vi "WindSensorSampleSensorLoop.vi"   [LabVIEW 2018]
uses:
  WindSensorSampleSensorLoopData.ctl
  WindSensorSampleSensorLoopStates.ctl
  WindSensorSample.ctl
  WindSensorErrorSample.ctl
  WindSensorErrorCodes.ctl
  <vilib>/Platform/TimedLoop/XDataNode/timing_clust.ctl
  <vilib>/Platform/TimedLoop/XDataNode/nitl_modes.ctl
  <vilib>/Platform/TimedLoop/XDataNode/wakeup.ctl
  <vilib>/rvi/Emulation/niFpgaSctlEmulationGetInTimedLoop.vi
  <vilib>/rvi/Emulation/niFpgaEmulationReportErrorSimple.vi
  <vilib>/rvi/Emulation/niFpgaGetClockAttributes.vi
  <vilib>/rvi/Emulation/niFpgaCriticalErrorInLSC.vi
  <vilib>/rvi/Emulation/niFpgaEmulationIsFPGAContextNoSignature.vi
  <vilib>/rvi/FIFO/Fifo_Resource/nirvififoEmulationSetSize.vi
  <vilib>/rvi/DataTransferAndStorage/Container/Common/niFpgaContainerGetUniqueNameForEmu.vi
  <vilib>/rvi/FIFO/Fifo_Resource/nirviFifoEmulationQueueMgr.vi
  <instcachedir>/0/nirviFifoEmulationQueueMgr_E5CAEC123FF24DC58D834DCA3CDAA9B5.lvgen/nirviFifoEmulationQueueMgr_E5CAEC123FF24DC58D834DCA3CDAA9B5_001.vi
  <vilib>/rvi/Emulation/niFpgaProcessEmulError.vi
  <vilib>/rvi/Memory/Memory_Emulation/niFpgaMemoryEmulationCacheClearOnFirstRun.vi
  <vilib>/rvi/Memory/Memory_Emulation/nirvimemoryEmulationManagerCache_MakeExclusive.vi
  <vilib>/rvi/Memory/Memory_Emulation/niFpgaMemoryEmulationValidateCache.vi
  <vilib>/rvi/Memory/Memory_Emulation/nirvimemoryEmulationManagerCache_InsertValue.vi
  <vilib>/Utility/error.llb/Clear Errors.vi
  <vilib>/rvi/Memory/Memory_Emulation/nirvimemoryEmulationManagerCache_ReleaseExclusive.vi
  <vilib>/rvi/Memory/Memory_Emulation/nirvimemoryEmulationManagerCache_GetValue.vi
  <vilib>/rvi/Memory/Memory_Emulation/nirvimemoryEmulationManagerCache_SetValue.vi
  <vilib>/rvi/errors/niFpgaSetErrorForExecOnDevCompSimple.vi
  <vilib>/rvi/eio/common/nirviEmuReportErrorAndStop.vi
  <instcachedir>/0/nirviFifoEmulationQueueMgr_E5CAEC123FF24DC58D834DCA3CDAA9B5.lvgen/nirviFifoEmulationQueueMgr_E5CAEC123FF24DC58D834DCA3CDAA9B5_002.vi
  <vilib>/rvi/FIFO/Fifo_Resource/nirvififoEmulationDetermineInputValidOut.vi
  <vilib>/rvi/FIFO/Fifo_Resource/nirvififoEmulationCreateLock.vi
  <vilib>/rvi/FIFO/Fifo_Resource/nirvififoEmulationObtainLock.vi
  <vilib>/rvi/FIFO/Fifo_Resource/nirvififoEmulationReleaseLock.vi
  <vilib>/rvi/occurrence/nirviWaitOnOccurrenceBase.vi
  <vilib>/rvi/errors/nirviReportUnexpectedCaseInternalError.vi
  <vilib>/rvi/errors/nirviReportUnexpectedCaseInternalError (U32).vi
  <instcachedir>/0/nirviFifoEmulationQueueMgr_E5CAEC123FF24DC58D834DCA3CDAA9B5.lvgen/nirviFifoEmulationQueueMgr_E5CAEC123FF24DC58D834DCA3CDAA9B5_004.vi
  <instcachedir>/0/nirviFifoEmulationQueueMgr_E5CAEC123FF24DC58D834DCA3CDAA9B5.lvgen/nirviFifoEmulationQueueMgr_E5CAEC123FF24DC58D834DCA3CDAA9B5_026.vi
  <instcachedir>/0/nirviFifoEmulationQueueMgr_E5CAEC123FF24DC58D834DCA3CDAA9B5.lvgen/nirviFifoEmulationQueueMgr_E5CAEC123FF24DC58D834DCA3CDAA9B5_027.vi
  <vilib>/Platform/TimedLoop/XDataNode/XDataNode.xnode
  <vilib>/rvi/DataTransferAndStorage/Container/XNode/niFpgaContainer.xnode
  <vilib>/rvi/FIFO/Fifo_Resource/nirvififoEmulationGetNumberOfElementsToRead.vi
  <vilib>/rvi/DataTransferAndStorage/Register/Emulation/niFpgaRegisterEmulation.vi
  <vilib>/rvi/FIFO/Fifo_Resource/nirvififoEmulationWrite.vi
  <vilib>/rvi/FIFO/Fifo_Resource/nirvififoEmulationRead.vi
  <vilib>/Platform/TimedLoop/XDataNode/XDNodeRunTimeDep.lvlib
types:
  T1 = typedef "WindSensorSampleSensorLoopData.ctl" = cluster{"State":T2, "StateAfterRead":T2, "Timestamp":u64, "U16":u16, "Negative":bool, "SGL":i32, "Timeout":i32, "Sample":T3, "ErrorSample":T4, "PushSignature":bool, "IgnoreComa":bool}
  T2 = typedef "WindSensorSampleSensorLoopStates.ctl" = enum16{"WaitForData", "StartX", "EndX", "StartY", "EndY", "StartZ", "EndZ", "StartT", "EndT", "StartD", "EndD", "StartC", "EndC", "StartS", "EndS", "CheckSignature", "ReadSGL", "ReadU16", "ReadHexU16", "PrepareSample", "MoveSample", "ResponseUnknownError", "ResponseInvalidError", "ResponseTimeoutError", "ResponseSignatureError", "PrepareErrorCode", "MoveErrorCode", "ClearRxFIFO", "WaitForClearComplete"}
  T3 = typedef "WindSensorSample.ctl" = cluster{"Timestamp":u64, "TxBytes":u64, "RxBytes":u64, "TxFrames":u64, "RxFrames":u64, "X":i32, "Y":i32, "Z":i32, "Temperature":i32, "DiagnosticWord":u16, "Count":u8, "Signature":u16}
  T4 = typedef "WindSensorErrorSample.ctl" = cluster{"Timestamp":u64, "TxBytes":u64, "RxBytes":u64, "TxFrames":u64, "RxFrames":u64, "ErrorCode":T5}
  T5 = typedef "WindSensorErrorCodes.ctl" = enum16{"None", "ResponseUnknownError", "ResponseInvalidError", "ResponseTimeoutError", "ResponseSignatureError"}
  T6 = typedef "XDNodeRunTimeDep.lvlib/timing_clust.ctl" = cluster{"Expected End [f-1]":u64, "Actual End [f-1]":u64, "Finished Late? [f-1]":bool, "Expected End [i-1]":u64, "Actual End [i-1]":u64, "Finished Late? [i-1]":bool, "Expected Start [i]":u64, "Actual Start [i]":u64, "Expected Start [f]":u64, "Actual Start [f]":u64, "Source Name":string, "Structure Name":string, "Period":i64, "Deadline":i64, "Offset":i64, "Start":i64, "Priority":i32, "Timeout":i32, "Mode":T7, "Wakeup Reason":T8, "Error":errorcluster, "Source Type":string, "Secondary Source Type":string, "Global End Time":u64, "Global Start Time":u64, "Frame Duration":u64, "Iteration Duration":u64, "Assigned CPU":i32, "I/O Scan Engine Mode":u32}
  T7 = typedef "XDNodeRunTimeDep.lvlib/nitl_modes.ctl" = enum32{"No Change", "Process missed periods, maintain original phase", "Discard missed periods, maintain original phase", "Process missed periods, ignore original phase", "Discard missed periods, ignore original phase"}
  T8 = typedef "XDNodeRunTimeDep.lvlib/wakeup.ctl" = enum32{"Normal", "Aborted", "Asynchronous wakeup", "Timing source error", "Timed loop error", "Timeout"}
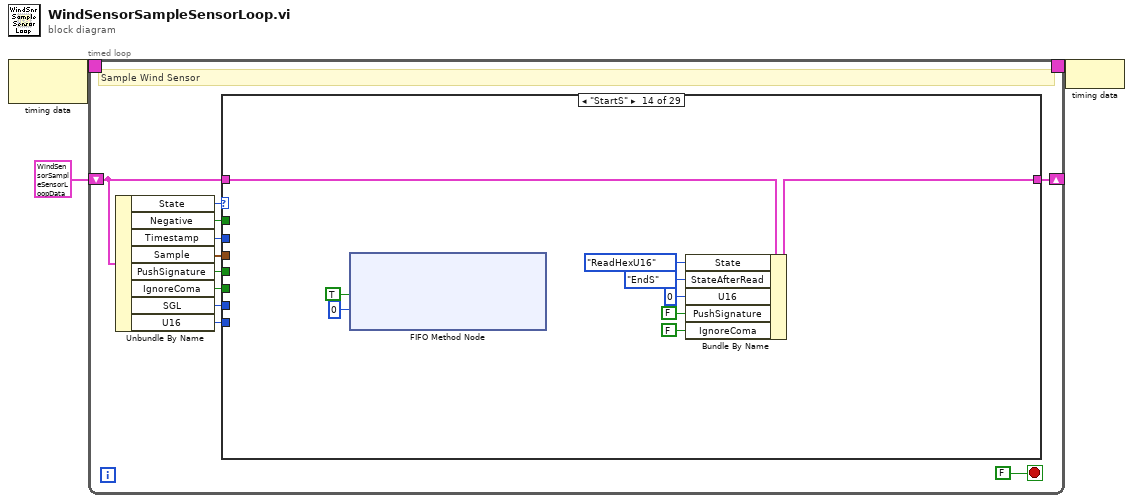
[diagram p0: block diagram]
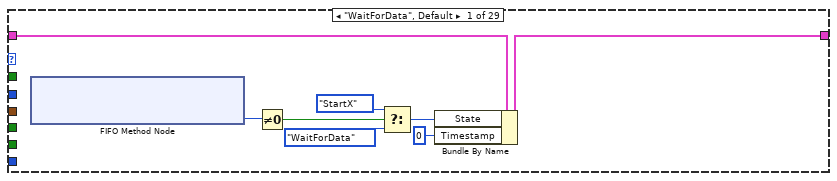
[diagram p2: hidden frame]
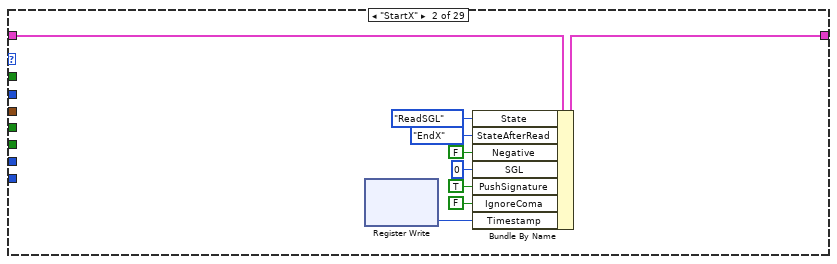
[diagram p3: hidden frame]
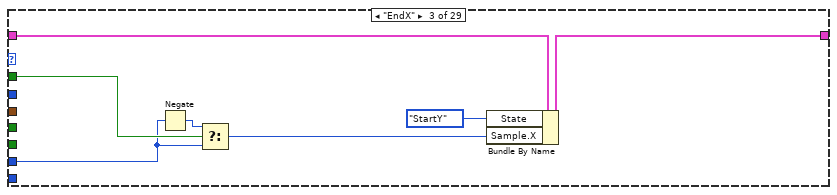
[diagram p4: hidden frame]
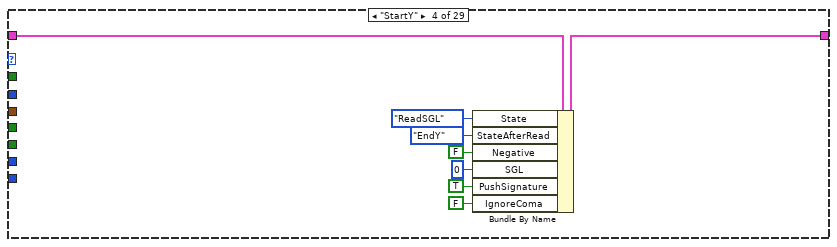
[diagram p5: hidden frame]
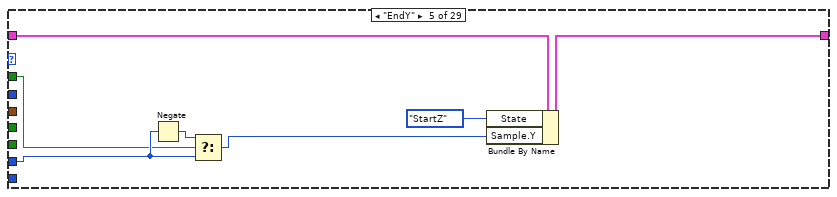
[diagram p6: hidden frame]
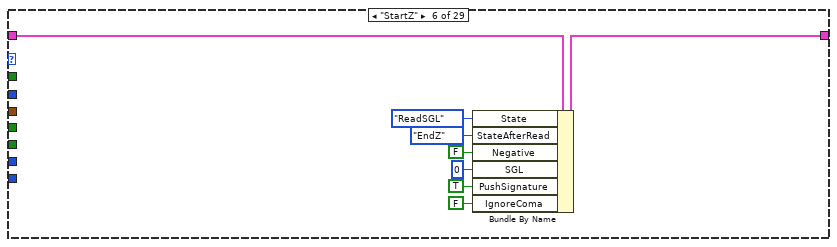
[diagram p7: hidden frame]
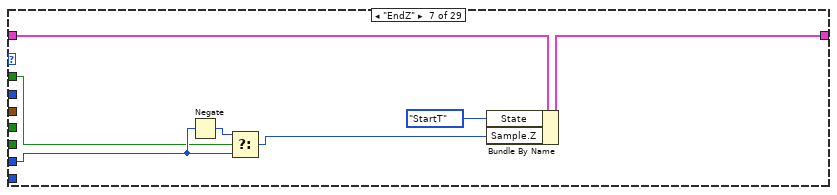
[diagram p8: hidden frame]
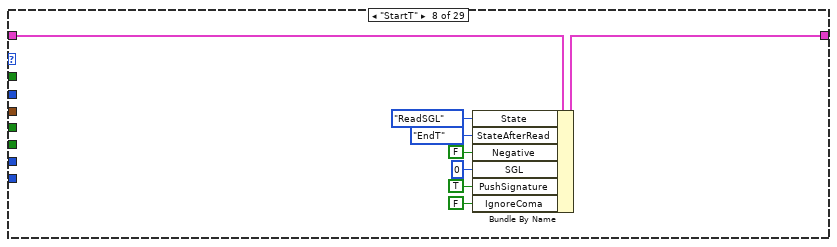
[diagram p9: hidden frame]
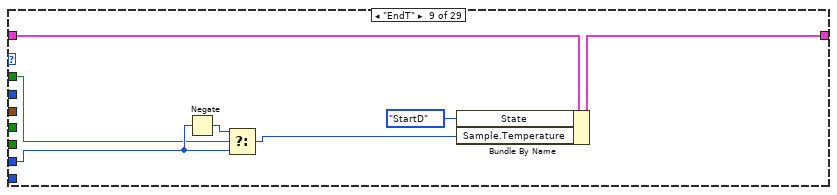
[diagram p10: hidden frame]
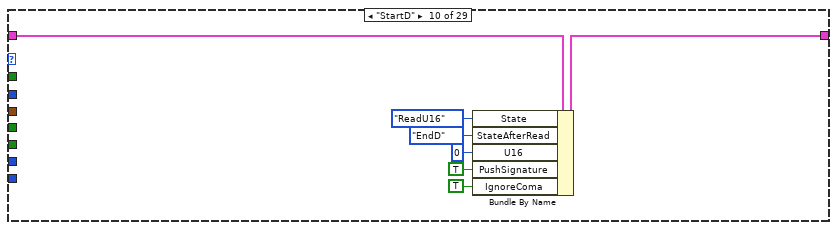
[diagram p11: hidden frame]
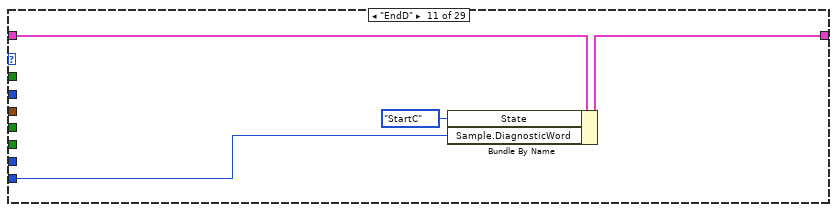
[diagram p12: hidden frame]
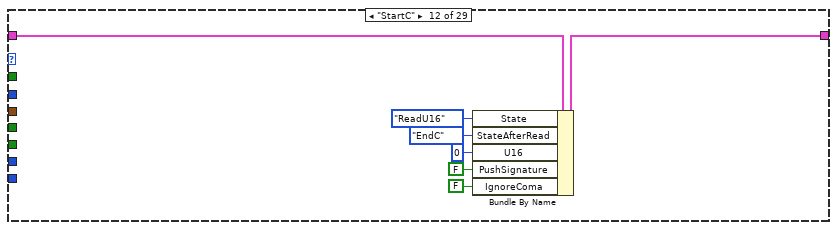
[diagram p13: hidden frame]
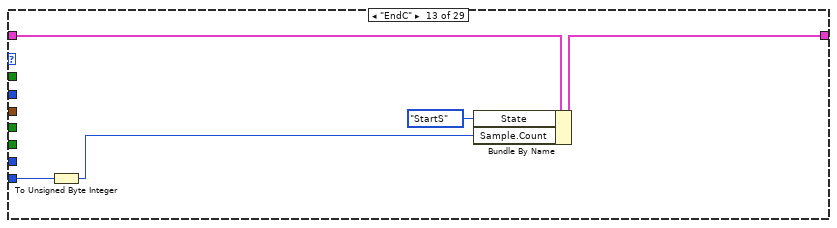
[diagram p14: hidden frame]
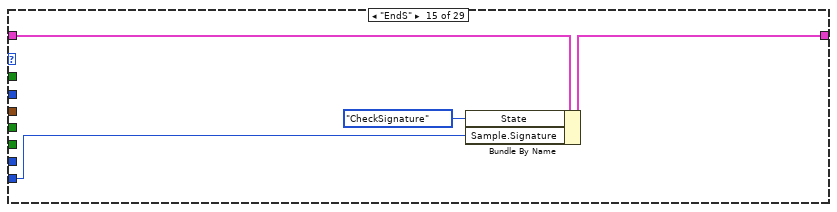
[diagram p15: hidden frame]
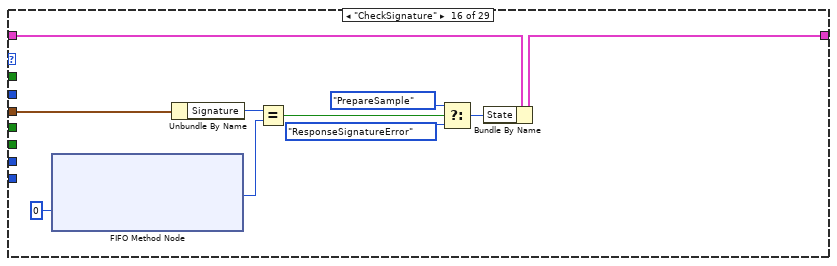
[diagram p16: hidden frame]
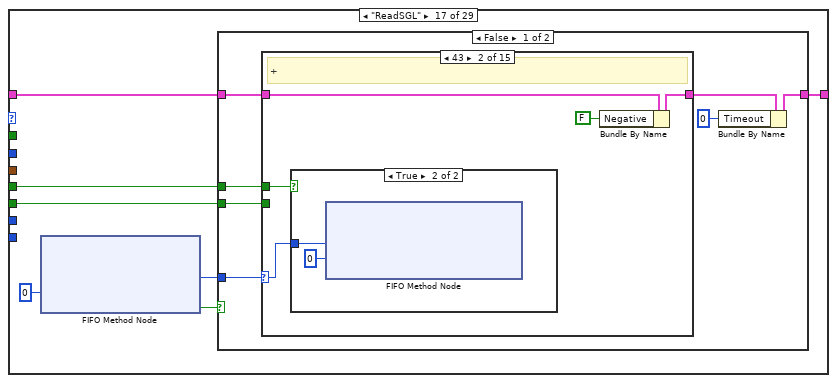
[diagram p17: hidden frame]
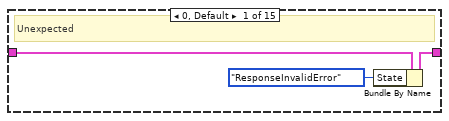
[diagram p18: hidden frame]
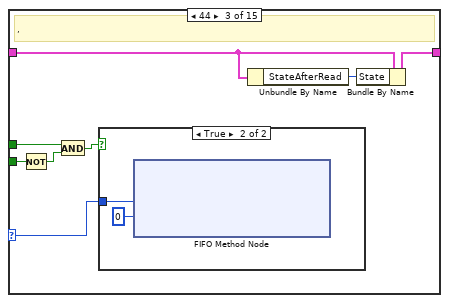
[diagram p20: hidden frame]
diagram:
  n1 = node-c288() -> (w3:T6)  [unwired: 1 in]
  n2 = timed-loop {
    timing: w3 -> [_]
    timing-out: [_] -> w2
    shift-right: [w14] -> _
    shift-left: T1 {"State"=enum."WaitForData", "StateAfterRead"=enum."WaitForData", "Timestamp"=0, "U16"=0, "Negative"=FALSE, "SGL"=0, "Timeout"=0, "Sample"={"Timestamp"=0, "TxBytes"=0, "RxBytes"=0, "TxFrames"=0, "RxFrames"=0, "X"=0, "Y"=0, "Z"=0, "Temperature"=0, "DiagnosticWord"=0, "Count"=0, "Signature"=0}, "ErrorSample"={"Timestamp"=0, "TxBytes"=0, "RxBytes"=0, "TxFrames"=0, "RxFrames"=0, "ErrorCode"=enum."None"}, "PushSignature"=FALSE, "IgnoreComa"=FALSE} ("DisplacementData") -> [w13]
    stop <- FALSE stop-if-true
    # "Sample Wind Sensor"
    n3 = Unbundle By Name(w13) -> ("State"=w12:T2, "Negative"=w11:bool, "Timestamp"=w9:u64, "Sample"=w10:T3, "PushSignature"=w7:bool, "IgnoreComa"=w6:bool, "SGL"=w5:i32, "U16"=w4:u16)
    n4 = case shown="\"StartS\"" w12 {
      tunnel: [w19 w30 w37 w45 w52 w60 w67 w75 w82 w89 w93 w100 w105 w114 w118 w123 w132 w286 w423 w558 w560 w566 w570 w574 w578 w588 w593 w598 w606] -> w14
      tunnel: w13 -> [w22 w31 w38 w46 w53 w61 w68 w76 w83 w90 w94 w101 w106 w115 w119 w124 w134 w292 w427 w559 w562 w568 w572 w576 w580 w584 w592 w597 w605]
      tunnel: w11 -> [_ _ w35 _ w47 _ w62 _ w77 _ _ _ _ _ _ _ _ _ _ _ _ _ _ _ _ _ _ _ _]
      tunnel: w10 -> [_ _ _ _ _ _ _ _ _ _ _ _ _ _ _ w128 _ _ _ _ w564 _ _ _ _ _ _ _ _]
      tunnel: w9 -> [_ _ _ _ _ _ _ _ _ _ _ _ _ _ _ _ _ _ _ w556 _ _ _ _ _ w583 _ _ _]
      tunnel: w7 -> [_ _ _ _ _ _ _ _ _ _ _ _ _ _ _ _ w131 w290 _ _ _ _ _ _ _ _ _ _ _]
      tunnel: w6 -> [_ _ _ _ _ _ _ _ _ _ _ _ _ _ _ _ w130 w289 _ _ _ _ _ _ _ _ _ _ _]
      tunnel: w5 -> [_ _ w33 _ w48 _ w64 _ w79 _ _ _ _ _ _ _ _ _ _ _ _ _ _ _ _ _ _ _ _]
      tunnel: w4 -> [_ _ _ _ _ _ _ _ _ _ w91 _ w103 _ w116 _ _ _ _ _ _ _ _ _ _ _ _ _ _]
      frame "WaitForData", Default {
        n5 = xnode ("FIFO Method Node")() -> ("Number of Elements to Read"=w17:u32)  [unwired: 1 in, 1 out]
        n6 = Not Equal To 0?(x=w17) -> (x != 0?=w16:bool)
        n7 = Select(t=WindSensorSampleSensorLoopStates."StartX" ("DisplacementStates"), s=w16, f=WindSensorSampleSensorLoopStates."WaitForData") -> (s? t:f=w20:T2)
        n8 = Bundle By Name(cluster=w22, "State"=w20, "Timestamp"=u64 0) -> (w19:T1)
      }
      frame "StartX" {
        n9 = xnode "Register Write"() -> ("Data"=w23:u64)  [unwired: 1 in, 1 out]
        n10 = Bundle By Name(cluster=w31, "State"=WindSensorSampleSensorLoopStates."ReadSGL", "StateAfterRead"=WindSensorSampleSensorLoopStates."EndX", "Negative"=FALSE, "SGL"=0, "PushSignature"=TRUE, "IgnoreComa"=FALSE, "Timestamp"=w23) -> (w30:T1)
      }
      frame "EndX" {
        n11 = Negate(x=w33) -> (-x=w34:i32)
        n12 = Select(t=w34, s=w35, f=w33) -> (s? t:f=w32:i32)
        n13 = Bundle By Name(cluster=w38, "State"=WindSensorSampleSensorLoopStates."StartY", "Sample.X"=w32) -> (w37:T1)
      }
      frame "StartY" {
        n14 = Bundle By Name(cluster=w46, "State"=WindSensorSampleSensorLoopStates."ReadSGL", "StateAfterRead"=WindSensorSampleSensorLoopStates."EndY", "Negative"=FALSE, "SGL"=0, "PushSignature"=TRUE, "IgnoreComa"=FALSE) -> (w45:T1)
      }
      frame "EndY" {
        n15 = Negate(x=w48) -> (-x=w50:i32)
        n16 = Select(t=w50, s=w47, f=w48) -> (s? t:f=w49:i32)
        n17 = Bundle By Name(cluster=w53, "State"=WindSensorSampleSensorLoopStates."StartZ", "Sample.Y"=w49) -> (w52:T1)
      }
      frame "StartZ" {
        n18 = Bundle By Name(cluster=w61, "State"=WindSensorSampleSensorLoopStates."ReadSGL", "StateAfterRead"=WindSensorSampleSensorLoopStates."EndZ", "Negative"=FALSE, "SGL"=0, "PushSignature"=TRUE, "IgnoreComa"=FALSE) -> (w60:T1)
      }
      frame "EndZ" {
        n19 = Negate(x=w64) -> (-x=w65:i32)
        n20 = Select(t=w65, s=w62, f=w64) -> (s? t:f=w63:i32)
        n21 = Bundle By Name(cluster=w68, "State"=WindSensorSampleSensorLoopStates."StartT", "Sample.Z"=w63) -> (w67:T1)
      }
      frame "StartT" {
        n22 = Bundle By Name(cluster=w76, "State"=WindSensorSampleSensorLoopStates."ReadSGL", "StateAfterRead"=WindSensorSampleSensorLoopStates."EndT", "Negative"=FALSE, "SGL"=0, "PushSignature"=TRUE, "IgnoreComa"=FALSE) -> (w75:T1)
      }
      frame "EndT" {
        n23 = Negate(x=w79) -> (-x=w80:i32)
        n24 = Select(t=w80, s=w77, f=w79) -> (s? t:f=w78:i32)
        n25 = Bundle By Name(cluster=w83, "State"=WindSensorSampleSensorLoopStates."StartD", "Sample.Temperature"=w78) -> (w82:T1)
      }
      frame "StartD" {
        n26 = Bundle By Name(cluster=w90, "State"=WindSensorSampleSensorLoopStates."ReadU16", "StateAfterRead"=WindSensorSampleSensorLoopStates."EndD", "U16"=u16 0, "PushSignature"=TRUE, "IgnoreComa"=TRUE) -> (w89:T1)
      }
      frame "EndD" {
        n27 = Bundle By Name(cluster=w94, "State"=WindSensorSampleSensorLoopStates."StartC", "Sample.DiagnosticWord"=w91) -> (w93:T1)
      }
      frame "StartC" {
        n28 = Bundle By Name(cluster=w101, "State"=WindSensorSampleSensorLoopStates."ReadU16", "StateAfterRead"=WindSensorSampleSensorLoopStates."EndC", "U16"=u16 0, "PushSignature"=FALSE, "IgnoreComa"=FALSE) -> (w100:T1)
      }
      frame "EndC" {
        n29 = To Unsigned Byte Integer(number=w103) -> (unsigned 8bit integer=w102:u8)
        n30 = Bundle By Name(cluster=w106, "State"=WindSensorSampleSensorLoopStates."StartS", "Sample.Count"=w102) -> (w105:T1)
      }
      frame "StartS" {
        n31 = xnode ("FIFO Method Node")("Element"=TRUE, "Timeout"=0) -> ()  [unwired: 1 in, 2 out]
        n32 = Bundle By Name(cluster=w115, "State"=WindSensorSampleSensorLoopStates."ReadHexU16", "StateAfterRead"=WindSensorSampleSensorLoopStates."EndS", "U16"=u16 0, "PushSignature"=FALSE, "IgnoreComa"=FALSE) -> (w114:T1)
      }
      frame "EndS" {
        n33 = Bundle By Name(cluster=w119, "State"=WindSensorSampleSensorLoopStates."CheckSignature", "Sample.Signature"=w116) -> (w118:T1)
      }
      frame "CheckSignature" {
        n34 = xnode ("FIFO Method Node")("Timeout"=0) -> ("Element"=w126:u16)  [unwired: 1 in, 2 out]
        n35 = Unbundle By Name(w128) -> ("Signature"=w127:u16)
        n36 = Equal?(x=w127, y=w126) -> (x = y?=w125:bool)
        n37 = Select(t=WindSensorSampleSensorLoopStates."PrepareSample" ("State"), s=w125, f=WindSensorSampleSensorLoopStates."ResponseSignatureError") -> (s? t:f=w120:T2)
        n38 = Bundle By Name(cluster=w124, "State"=w120) -> (w123:T1)
      }
      frame "ReadSGL" {
        n39 = xnode ("FIFO Method Node")("Timeout"=0) -> ("Element"=w133:u8, "Timed Out?"=w135:bool)  [unwired: 1 in, 1 out]
        n40 = case shown="False" w135 {
          tunnel: w134 -> [w143 w285]
          tunnel: [w138 w284] -> w132
          tunnel: w133 -> [w142 _]
          tunnel: w131 -> [w141 _]
          tunnel: w130 -> [w140 _]
          frame False {
            n41 = case shown="43" w142 {
              selector: w142 -> [_ w147 w158 w164 w171 w176 w185 w196 w207 w218 w229 w240 w251 w262 w273]
              tunnel: w143 -> [w146 w151 w160 w167 w173 w181 w192 w203 w214 w225 w236 w247 w258 w269 w280]
              tunnel: [w145 w150 w161 w168 w173 w182 w193 w204 w215 w226 w237 w248 w259 w270 w281] -> w139
              tunnel: w141 -> [_ w148 w156 w165 w172 w177 w186 w197 w208 w219 w230 w241 w252 w263 w274]
              tunnel: w140 -> [_ _ w154 _ _ _ _ _ _ _ _ _ _ _ _]
              frame 0, Default {
                # "Unexpected"
                n42 = Bundle By Name(cluster=w146, "State"=WindSensorSampleSensorLoopStates."ResponseInvalidError") -> (w145:T1)
              }
              frame 43 {
                # "+"
                n43 = case shown="True" w148 {
                  tunnel: w147 -> [_ w153]
                  frame False {
                  }
                  frame True {
                    n44 = xnode ("FIFO Method Node")("Element"=w153, "Timeout"=0) -> ()  [unwired: 1 in, 2 out]
                  }
                }
                n45 = Bundle By Name(cluster=w151, "Negative"=FALSE) -> (w150:T1)
              }
              frame 44 {
                # ","
                n46 = Not(x=w154) -> (.not. x?=w157:bool)
                n47 = And(x=w156, y=w157) -> (x .and. y?=w155:bool)
                n48 = case shown="True" w155 {
                  tunnel: w158 -> [_ w163]
                  frame False {
                  }
                  frame True {
                    n49 = xnode ("FIFO Method Node")("Element"=w163, "Timeout"=0) -> ()  [unwired: 1 in, 2 out]
                  }
                }
                n50 = Unbundle By Name(w160) -> ("StateAfterRead"=w159:T2)
                n51 = Bundle By Name(cluster=w160, "State"=w159) -> (w161:T1)
              }
              frame 45 {
                # "-"
                n52 = case shown="True" w165 {
                  tunnel: w164 -> [_ w170]
                  frame False {
                  }
                  frame True {
                    n53 = xnode ("FIFO Method Node")("Element"=w170, "Timeout"=0) -> ()  [unwired: 1 in, 2 out]
                  }
                }
                n54 = Bundle By Name(cluster=w167, "Negative"=TRUE) -> (w168:T1)
              }
              frame 46 {
                # "."
                n55 = case shown="True" w172 {
                  tunnel: w171 -> [_ w175]
                  frame False {
                  }
                  frame True {
                    n56 = xnode ("FIFO Method Node")("Element"=w175, "Timeout"=0) -> ()  [unwired: 1 in, 2 out]
                  }
                }
              }
              frame 48 {
                # "0"
                n57 = case shown="True" w177 {
                  tunnel: w176 -> [_ w184]
                  frame False {
                  }
                  frame True {
                    n58 = xnode ("FIFO Method Node")("Element"=w184, "Timeout"=0) -> ()  [unwired: 1 in, 2 out]
                  }
                }
                n59 = Unbundle By Name(w181) -> ("SGL"=w180:i32)
                n60 = Multiply(x=w180, y=10) -> (x*y=w178:i32)
                n61 = Bundle By Name(cluster=w181, "SGL"=w178) -> (w182:T1)
              }
              frame 49 {
                # "1"
                n62 = case shown="True" w186 {
                  tunnel: w185 -> [_ w195]
                  frame False {
                  }
                  frame True {
                    n63 = xnode ("FIFO Method Node")("Element"=w195, "Timeout"=0) -> ()  [unwired: 1 in, 2 out]
                  }
                }
                n64 = Unbundle By Name(w192) -> ("SGL"=w191:i32)
                n65 = Multiply(x=w191, y=10) -> (x*y=w189:i32)
                n66 = Add(x=w189, y=1) -> (x+y=w188:i32)
                n67 = Bundle By Name(cluster=w192, "SGL"=w188) -> (w193:T1)
              }
              frame 50 {
                # "2"
                n68 = case shown="True" w197 {
                  tunnel: w196 -> [_ w206]
                  frame False {
                  }
                  frame True {
                    n69 = xnode ("FIFO Method Node")("Element"=w206, "Timeout"=0) -> ()  [unwired: 1 in, 2 out]
                  }
                }
                n70 = Unbundle By Name(w203) -> ("SGL"=w202:i32)
                n71 = Multiply(x=w202, y=10) -> (x*y=w200:i32)
                n72 = Add(x=w200, y=2) -> (x+y=w199:i32)
                n73 = Bundle By Name(cluster=w203, "SGL"=w199) -> (w204:T1)
              }
              frame 51 {
                # "3"
                n74 = case shown="True" w208 {
                  tunnel: w207 -> [_ w217]
                  frame False {
                  }
                  frame True {
                    n75 = xnode ("FIFO Method Node")("Element"=w217, "Timeout"=0) -> ()  [unwired: 1 in, 2 out]
                  }
                }
                n76 = Unbundle By Name(w214) -> ("SGL"=w213:i32)
                n77 = Multiply(x=w213, y=10) -> (x*y=w211:i32)
                n78 = Add(x=w211, y=3) -> (x+y=w210:i32)
                n79 = Bundle By Name(cluster=w214, "SGL"=w210) -> (w215:T1)
              }
              frame 52 {
                # "4"
                n80 = case shown="True" w219 {
                  tunnel: w218 -> [_ w228]
                  frame False {
                  }
                  frame True {
                    n81 = xnode ("FIFO Method Node")("Element"=w228, "Timeout"=0) -> ()  [unwired: 1 in, 2 out]
                  }
                }
                n82 = Unbundle By Name(w225) -> ("SGL"=w224:i32)
                n83 = Multiply(x=w224, y=10) -> (x*y=w222:i32)
                n84 = Add(x=w222, y=4) -> (x+y=w221:i32)
                n85 = Bundle By Name(cluster=w225, "SGL"=w221) -> (w226:T1)
              }
              frame 53 {
                # "5"
                n86 = case shown="True" w230 {
                  tunnel: w229 -> [_ w239]
                  frame False {
                  }
                  frame True {
                    n87 = xnode ("FIFO Method Node")("Element"=w239, "Timeout"=0) -> ()  [unwired: 1 in, 2 out]
                  }
                }
                n88 = Unbundle By Name(w236) -> ("SGL"=w235:i32)
                n89 = Multiply(x=w235, y=10) -> (x*y=w233:i32)
                n90 = Add(x=w233, y=5) -> (x+y=w232:i32)
                n91 = Bundle By Name(cluster=w236, "SGL"=w232) -> (w237:T1)
              }
              frame 54 {
                # "6"
                n92 = case shown="True" w241 {
                  tunnel: w240 -> [_ w250]
                  frame False {
                  }
                  frame True {
                    n93 = xnode ("FIFO Method Node")("Element"=w250, "Timeout"=0) -> ()  [unwired: 1 in, 2 out]
                  }
                }
                n94 = Unbundle By Name(w247) -> ("SGL"=w246:i32)
                n95 = Multiply(x=w246, y=10) -> (x*y=w244:i32)
                n96 = Add(x=w244, y=6) -> (x+y=w243:i32)
                n97 = Bundle By Name(cluster=w247, "SGL"=w243) -> (w248:T1)
              }
              frame 55 {
                # "7"
                n98 = case shown="True" w252 {
                  tunnel: w251 -> [_ w261]
                  frame False {
                  }
                  frame True {
                    n99 = xnode ("FIFO Method Node")("Element"=w261, "Timeout"=0) -> ()  [unwired: 1 in, 2 out]
                  }
                }
                n100 = Unbundle By Name(w258) -> ("SGL"=w257:i32)
                n101 = Multiply(x=w257, y=10) -> (x*y=w255:i32)
                n102 = Add(x=w255, y=7) -> (x+y=w254:i32)
                n103 = Bundle By Name(cluster=w258, "SGL"=w254) -> (w259:T1)
              }
              frame 56 {
                # "8"
                n104 = case shown="True" w263 {
                  tunnel: w262 -> [_ w272]
                  frame False {
                  }
                  frame True {
                    n105 = xnode ("FIFO Method Node")("Element"=w272, "Timeout"=0) -> ()  [unwired: 1 in, 2 out]
                  }
                }
                n106 = Unbundle By Name(w269) -> ("SGL"=w268:i32)
                n107 = Multiply(x=w268, y=10) -> (x*y=w266:i32)
                n108 = Add(x=w266, y=8) -> (x+y=w265:i32)
                n109 = Bundle By Name(cluster=w269, "SGL"=w265) -> (w270:T1)
              }
              frame 57 {
                # "9"
                n110 = case shown="True" w274 {
                  tunnel: w273 -> [_ w283]
                  frame False {
                  }
                  frame True {
                    n111 = xnode ("FIFO Method Node")("Element"=w283, "Timeout"=0) -> ()  [unwired: 1 in, 2 out]
                  }
                }
                n112 = Unbundle By Name(w280) -> ("SGL"=w279:i32)
                n113 = Multiply(x=w279, y=10) -> (x*y=w277:i32)
                n114 = Add(x=w277, y=9) -> (x+y=w276:i32)
                n115 = Bundle By Name(cluster=w280, "SGL"=w276) -> (w281:T1)
              }
            }
            n116 = Bundle By Name(cluster=w139, "Timeout"=0) -> (w138:T1)
          }
          frame True {
            n117 = call "WindSensorCheckForTimeout.vi"("WindSensorSampleSensorLoopData in"=w285) -> ("WindSensorSampleSensorLoopData out"=w284:T1)  [unwired: 10 in]
          }
        }
      }
      frame "ReadU16" {
        n118 = xnode ("FIFO Method Node")("Timeout"=0) -> ("Element"=w291:u8, "Timed Out?"=w293:bool)  [unwired: 1 in, 1 out]
        n119 = case shown="False" w293 {
          tunnel: w292 -> [w299 w422]
          tunnel: [w298 w421] -> w287
          tunnel: w291 -> [w297 _]
          tunnel: w290 -> [w296 _]
          tunnel: w289 -> [w295 _]
          frame False {
            n120 = case shown="0, Default" w297 {
              selector: w297 -> [_ w303 w313 w322 w333 w344 w355 w366 w377 w388 w399 w410]
              tunnel: w299 -> [w302 w309 w318 w329 w340 w351 w362 w373 w384 w395 w406 w417]
              tunnel: [w301 w310 w319 w330 w341 w352 w363 w374 w385 w396 w407 w418] -> w298
              tunnel: w296 -> [_ w306 w314 w323 w334 w345 w356 w367 w378 w389 w400 w411]
              tunnel: w295 -> [_ w305 _ _ _ _ _ _ _ _ _ _]
              frame 0, Default {
                # "Unexpected"
                n121 = Bundle By Name(cluster=w302, "State"=WindSensorSampleSensorLoopStates."ResponseInvalidError") -> (w301:T1)
              }
              frame 44 {
                # ","
                n122 = Not(x=w305) -> (.not. x?=w307:bool)
                n123 = And(x=w306, y=w307) -> (x .and. y?=w304:bool)
                n124 = case shown="True" w304 {
                  tunnel: w303 -> [_ w312]
                  frame False {
                  }
                  frame True {
                    n125 = xnode ("FIFO Method Node")("Element"=w312, "Timeout"=0) -> ()  [unwired: 1 in, 2 out]
                  }
                }
                n126 = Unbundle By Name(w309) -> ("StateAfterRead"=w308:T2)
                n127 = Bundle By Name(cluster=w309, "State"=w308) -> (w310:T1)
              }
              frame 48 {
                # "0"
                n128 = case shown="True" w314 {
                  tunnel: w313 -> [_ w321]
                  frame False {
                  }
                  frame True {
                    n129 = xnode ("FIFO Method Node")("Element"=w321, "Timeout"=0) -> ()  [unwired: 1 in, 2 out]
                  }
                }
                n130 = Unbundle By Name(w318) -> ("U16"=w317:u16)
                n131 = Multiply(x=w317, y=u16 10) -> (x*y=w315:u16)
                n132 = Bundle By Name(cluster=w318, "U16"=w315) -> (w319:T1)
              }
              frame 49 {
                # "1"
                n133 = case shown="True" w323 {
                  tunnel: w322 -> [_ w332]
                  frame False {
                  }
                  frame True {
                    n134 = xnode ("FIFO Method Node")("Element"=w332, "Timeout"=0) -> ()  [unwired: 1 in, 2 out]
                  }
                }
                n135 = Unbundle By Name(w329) -> ("U16"=w328:u16)
                n136 = Multiply(x=w328, y=u16 10) -> (x*y=w326:u16)
                n137 = Add(x=w326, y=u16 1) -> (x+y=w325:u16)
                n138 = Bundle By Name(cluster=w329, "U16"=w325) -> (w330:T1)
              }
              frame 50 {
                # "2"
                n139 = case shown="True" w334 {
                  tunnel: w333 -> [_ w343]
                  frame False {
                  }
                  frame True {
                    n140 = xnode ("FIFO Method Node")("Element"=w343, "Timeout"=0) -> ()  [unwired: 1 in, 2 out]
                  }
                }
                n141 = Unbundle By Name(w340) -> ("U16"=w339:u16)
                n142 = Multiply(x=w339, y=u16 10) -> (x*y=w337:u16)
                n143 = Add(x=w337, y=u16 2) -> (x+y=w336:u16)
                n144 = Bundle By Name(cluster=w340, "U16"=w336) -> (w341:T1)
              }
              frame 51 {
                # "3"
                n145 = case shown="True" w345 {
                  tunnel: w344 -> [_ w354]
                  frame False {
                  }
                  frame True {
                    n146 = xnode ("FIFO Method Node")("Element"=w354, "Timeout"=0) -> ()  [unwired: 1 in, 2 out]
                  }
                }
                n147 = Unbundle By Name(w351) -> ("U16"=w350:u16)
                n148 = Multiply(x=w350, y=u16 10) -> (x*y=w348:u16)
                n149 = Add(x=w348, y=u16 3) -> (x+y=w347:u16)
                n150 = Bundle By Name(cluster=w351, "U16"=w347) -> (w352:T1)
              }
              frame 52 {
                # "4"
                n151 = case shown="True" w356 {
                  tunnel: w355 -> [_ w365]
                  frame False {
                  }
                  frame True {
                    n152 = xnode ("FIFO Method Node")("Element"=w365, "Timeout"=0) -> ()  [unwired: 1 in, 2 out]
                  }
                }
                n153 = Unbundle By Name(w362) -> ("U16"=w361:u16)
                n154 = Multiply(x=w361, y=u16 10) -> (x*y=w359:u16)
                n155 = Add(x=w359, y=u16 4) -> (x+y=w358:u16)
                n156 = Bundle By Name(cluster=w362, "U16"=w358) -> (w363:T1)
              }
              frame 53 {
                # "5"
                n157 = case shown="True" w367 {
                  tunnel: w366 -> [_ w376]
                  frame False {
                  }
                  frame True {
                    n158 = xnode ("FIFO Method Node")("Element"=w376, "Timeout"=0) -> ()  [unwired: 1 in, 2 out]
                  }
                }
                n159 = Unbundle By Name(w373) -> ("U16"=w372:u16)
                n160 = Multiply(x=w372, y=u16 10) -> (x*y=w370:u16)
                n161 = Add(x=w370, y=u16 5) -> (x+y=w369:u16)
                n162 = Bundle By Name(cluster=w373, "U16"=w369) -> (w374:T1)
              }
              frame 54 {
                # "6"
                n163 = case shown="True" w378 {
                  tunnel: w377 -> [_ w387]
                  frame False {
                  }
                  frame True {
                    n164 = xnode ("FIFO Method Node")("Element"=w387, "Timeout"=0) -> ()  [unwired: 1 in, 2 out]
                  }
                }
                n165 = Unbundle By Name(w384) -> ("U16"=w383:u16)
                n166 = Multiply(x=w383, y=u16 10) -> (x*y=w381:u16)
                n167 = Add(x=w381, y=u16 6) -> (x+y=w380:u16)
                n168 = Bundle By Name(cluster=w384, "U16"=w380) -> (w385:T1)
              }
              frame 55 {
                # "7"
                n169 = case shown="True" w389 {
                  tunnel: w388 -> [_ w398]
                  frame False {
                  }
                  frame True {
                    n170 = xnode ("FIFO Method Node")("Element"=w398, "Timeout"=0) -> ()  [unwired: 1 in, 2 out]
                  }
                }
                n171 = Unbundle By Name(w395) -> ("U16"=w394:u16)
                n172 = Multiply(x=w394, y=u16 10) -> (x*y=w392:u16)
                n173 = Add(x=w392, y=u16 7) -> (x+y=w391:u16)
                n174 = Bundle By Name(cluster=w395, "U16"=w391) -> (w396:T1)
              }
              frame 56 {
                # "8"
                n175 = case shown="True" w400 {
                  tunnel: w399 -> [_ w409]
                  frame False {
                  }
                  frame True {
                    n176 = xnode ("FIFO Method Node")("Element"=w409, "Timeout"=0) -> ()  [unwired: 1 in, 2 out]
                  }
                }
                n177 = Unbundle By Name(w406) -> ("U16"=w405:u16)
                n178 = Multiply(x=w405, y=u16 10) -> (x*y=w403:u16)
                n179 = Add(x=w403, y=u16 8) -> (x+y=w402:u16)
                n180 = Bundle By Name(cluster=w406, "U16"=w402) -> (w407:T1)
              }
              frame 57 {
                # "9"
                n181 = case shown="True" w411 {
                  tunnel: w410 -> [_ w420]
                  frame False {
                  }
                  frame True {
                    n182 = xnode ("FIFO Method Node")("Element"=w420, "Timeout"=0) -> ()  [unwired: 1 in, 2 out]
                  }
                }
                n183 = Unbundle By Name(w417) -> ("U16"=w416:u16)
                n184 = Multiply(x=w416, y=u16 10) -> (x*y=w414:u16)
                n185 = Add(x=w414, y=u16 9) -> (x+y=w413:u16)
                n186 = Bundle By Name(cluster=w417, "U16"=w413) -> (w418:T1)
              }
            }
          }
          frame True {
            n187 = call "WindSensorCheckForTimeout.vi"("WindSensorSampleSensorLoopData in"=w422) -> ("WindSensorSampleSensorLoopData out"=w421:T1)  [unwired: 10 in]
          }
        }
        n188 = Bundle By Name(cluster=w287, "Timeout"=0) -> (w286:T1)
      }
      frame "ReadHexU16" {
        n189 = xnode ("FIFO Method Node")("Timeout"=0) -> ("Element"=w426:u8, "Timed Out?"=w428:bool)  [unwired: 1 in, 1 out]
        n190 = case shown="False" w428 {
          tunnel: w427 -> [w432 w550]
          tunnel: [w431 w549] -> w424
          tunnel: w426 -> [w430 _]
          frame False {
            n191 = case shown="13" w430 {
              tunnel: w432 -> [w435 w437 w442 w449 w456 w463 w470 w477 w484 w491 w498 w505 w512 w519 w526 w533 w540 w547]
              tunnel: [w434 w438 w443 w450 w457 w464 w471 w478 w485 w492 w499 w506 w513 w520 w527 w534 w541 w548] -> w431
              frame 0, Default {
                # "Unexpected"
                n192 = Bundle By Name(cluster=w435, "State"=WindSensorSampleSensorLoopStates."ResponseInvalidError") -> (w434:T1)
              }
              frame 13 {
                # "\\r"
                n193 = Unbundle By Name(w437) -> ("StateAfterRead"=w436:T2)
                n194 = Bundle By Name(cluster=w437, "State"=w436) -> (w438:T1)
              }
              frame 48 {
                # "0"
                n195 = Unbundle By Name(w442) -> ("U16"=w441:u16)
                n196 = Multiply(x=w441, y=u16 16) -> (x*y=w439:u16)
                n197 = Bundle By Name(cluster=w442, "U16"=w439) -> (w443:T1)
              }
              frame 49 {
                # "1"
                n198 = Unbundle By Name(w449) -> ("U16"=w448:u16)
                n199 = Multiply(x=w448, y=u16 16) -> (x*y=w446:u16)
                n200 = Add(x=w446, y=u16 1) -> (x+y=w445:u16)
                n201 = Bundle By Name(cluster=w449, "U16"=w445) -> (w450:T1)
              }
              frame 50 {
                # "2"
                n202 = Unbundle By Name(w456) -> ("U16"=w455:u16)
                n203 = Multiply(x=w455, y=u16 16) -> (x*y=w453:u16)
                n204 = Add(x=w453, y=u16 2) -> (x+y=w452:u16)
                n205 = Bundle By Name(cluster=w456, "U16"=w452) -> (w457:T1)
              }
              frame 51 {
                # "3"
                n206 = Unbundle By Name(w463) -> ("U16"=w462:u16)
                n207 = Multiply(x=w462, y=u16 16) -> (x*y=w460:u16)
                n208 = Add(x=w460, y=u16 3) -> (x+y=w459:u16)
                n209 = Bundle By Name(cluster=w463, "U16"=w459) -> (w464:T1)
              }
              frame 52 {
                # "4"
                n210 = Unbundle By Name(w470) -> ("U16"=w469:u16)
                n211 = Multiply(x=w469, y=u16 16) -> (x*y=w467:u16)
                n212 = Add(x=w467, y=u16 4) -> (x+y=w466:u16)
                n213 = Bundle By Name(cluster=w470, "U16"=w466) -> (w471:T1)
              }
              frame 53 {
                # "5"
                n214 = Unbundle By Name(w477) -> ("U16"=w476:u16)
                n215 = Multiply(x=w476, y=u16 16) -> (x*y=w474:u16)
                n216 = Add(x=w474, y=u16 5) -> (x+y=w473:u16)
                n217 = Bundle By Name(cluster=w477, "U16"=w473) -> (w478:T1)
              }
              frame 54 {
                # "6"
                n218 = Unbundle By Name(w484) -> ("U16"=w483:u16)
                n219 = Multiply(x=w483, y=u16 16) -> (x*y=w481:u16)
                n220 = Add(x=w481, y=u16 6) -> (x+y=w480:u16)
                n221 = Bundle By Name(cluster=w484, "U16"=w480) -> (w485:T1)
              }
              frame 55 {
                # "7"
                n222 = Unbundle By Name(w491) -> ("U16"=w490:u16)
                n223 = Multiply(x=w490, y=u16 16) -> (x*y=w488:u16)
                n224 = Add(x=w488, y=u16 7) -> (x+y=w487:u16)
                n225 = Bundle By Name(cluster=w491, "U16"=w487) -> (w492:T1)
              }
              frame 56 {
                # "8"
                n226 = Unbundle By Name(w498) -> ("U16"=w497:u16)
                n227 = Multiply(x=w497, y=u16 16) -> (x*y=w495:u16)
                n228 = Add(x=w495, y=u16 8) -> (x+y=w494:u16)
                n229 = Bundle By Name(cluster=w498, "U16"=w494) -> (w499:T1)
              }
              frame 57 {
                # "9"
                n230 = Unbundle By Name(w505) -> ("U16"=w504:u16)
                n231 = Multiply(x=w504, y=u16 16) -> (x*y=w502:u16)
                n232 = Add(x=w502, y=u16 9) -> (x+y=w501:u16)
                n233 = Bundle By Name(cluster=w505, "U16"=w501) -> (w506:T1)
              }
              frame 97 {
                # "a"
                n234 = Unbundle By Name(w512) -> ("U16"=w511:u16)
                n235 = Multiply(x=w511, y=u16 16) -> (x*y=w509:u16)
                n236 = Add(x=w509, y=u16 10) -> (x+y=w508:u16)
                n237 = Bundle By Name(cluster=w512, "U16"=w508) -> (w513:T1)
              }
              frame 98 {
                # "b"
                n238 = Unbundle By Name(w519) -> ("U16"=w518:u16)
                n239 = Multiply(x=w518, y=u16 16) -> (x*y=w516:u16)
                n240 = Add(x=w516, y=u16 11) -> (x+y=w515:u16)
                n241 = Bundle By Name(cluster=w519, "U16"=w515) -> (w520:T1)
              }
              frame 99 {
                # "c"
                n242 = Unbundle By Name(w526) -> ("U16"=w525:u16)
                n243 = Multiply(x=w525, y=u16 16) -> (x*y=w523:u16)
                n244 = Add(x=w523, y=u16 12) -> (x+y=w522:u16)
                n245 = Bundle By Name(cluster=w526, "U16"=w522) -> (w527:T1)
              }
              frame 100 {
                # "d"
                n246 = Unbundle By Name(w533) -> ("U16"=w532:u16)
                n247 = Multiply(x=w532, y=u16 16) -> (x*y=w530:u16)
                n248 = Add(x=w530, y=u16 13) -> (x+y=w529:u16)
                n249 = Bundle By Name(cluster=w533, "U16"=w529) -> (w534:T1)
              }
              frame 101 {
                # "e"
                n250 = Unbundle By Name(w540) -> ("U16"=w539:u16)
                n251 = Multiply(x=w539, y=u16 16) -> (x*y=w537:u16)
                n252 = Add(x=w537, y=u16 14) -> (x+y=w536:u16)
                n253 = Bundle By Name(cluster=w540, "U16"=w536) -> (w541:T1)
              }
              frame 102 {
                # "f"
                n254 = Unbundle By Name(w547) -> ("U16"=w546:u16)
                n255 = Multiply(x=w546, y=u16 16) -> (x*y=w544:u16)
                n256 = Add(x=w544, y=u16 15) -> (x+y=w543:u16)
                n257 = Bundle By Name(cluster=w547, "U16"=w543) -> (w548:T1)
              }
            }
          }
          frame True {
            n258 = call "WindSensorCheckForTimeout.vi"("WindSensorSampleSensorLoopData in"=w550) -> ("WindSensorSampleSensorLoopData out"=w549:T1)  [unwired: 10 in]
          }
        }
        n259 = Bundle By Name(cluster=w424, "Timeout"=0) -> (w423:T1)
      }
      frame "PrepareSample" {
        n260 = xnode "Register Write"() -> ("Data"=w552:u64)  [unwired: 1 in, 1 out]
        n261 = xnode "Register Write"() -> ("Data"=w553:u64)  [unwired: 1 in, 1 out]
        n262 = xnode "Register Write"() -> ("Data"=w555:u64)  [unwired: 1 in, 1 out]
        n263 = xnode "Register Write"() -> ("Data"=w554:u64)  [unwired: 1 in, 1 out]
        n264 = Increment(x=w552) -> (x+1=w551:u64)
        n265 = xnode "Register Write"("Data"=w551) -> ()  [unwired: 1 in, 1 out]
        n266 = Bundle By Name(cluster=w559, "State"=WindSensorSampleSensorLoopStates."MoveSample", "Sample.Timestamp"=w556, "Sample.RxFrames"=w551, "Sample.TxBytes"=w555, "Sample.RxBytes"=w554, "Sample.TxFrames"=w553) -> (w558:T1)
      }
      frame "MoveSample" {
        n267 = xnode ("FIFO Method Node")("Element"=w564, "Timeout"=0) -> ()  [unwired: 1 in, 2 out]
        n268 = Bundle By Name(cluster=w562, "State"=WindSensorSampleSensorLoopStates."WaitForData") -> (w560:T1)
      }
      frame "ResponseUnknownError" {
        n269 = Bundle By Name(cluster=w568, "State"=WindSensorSampleSensorLoopStates."PrepareErrorCode", "ErrorSample.ErrorCode"=WindSensorErrorCodes."ResponseUnknownError") -> (w566:T1)
      }
      frame "ResponseInvalidError" {
        n270 = Bundle By Name(cluster=w572, "State"=WindSensorSampleSensorLoopStates."PrepareErrorCode", "ErrorSample.ErrorCode"=WindSensorErrorCodes."ResponseInvalidError") -> (w570:T1)
      }
      frame "ResponseTimeoutError" {
        n271 = Bundle By Name(cluster=w576, "State"=WindSensorSampleSensorLoopStates."PrepareErrorCode", "ErrorSample.ErrorCode"=WindSensorErrorCodes."ResponseTimeoutError") -> (w574:T1)
      }
      frame "ResponseSignatureError" {
        n272 = Bundle By Name(cluster=w580, "State"=WindSensorSampleSensorLoopStates."PrepareErrorCode", "ErrorSample.ErrorCode"=WindSensorErrorCodes."ResponseSignatureError") -> (w578:T1)
      }
      frame "PrepareErrorCode" {
        n273 = xnode "Register Write"() -> ("Data"=w582:u64)  [unwired: 1 in, 1 out]
        n274 = xnode "Register Read"() -> ("Data"=w586:u64)  [unwired: 1 in, 1 out]
        n275 = xnode "Register Read"() -> ("Data"=w585:u64)  [unwired: 1 in, 1 out]
        n276 = xnode "Register Read"() -> ("Data"=w587:u64)  [unwired: 1 in, 1 out]
        n277 = Increment(x=w582) -> (x+1=w581:u64)
        n278 = xnode "Register Write"("Data"=w581) -> ()  [unwired: 1 in, 1 out]
        n279 = Bundle By Name(cluster=w584, "State"=WindSensorSampleSensorLoopStates."MoveErrorCode", "ErrorSample.RxFrames"=w581, "ErrorSample.Timestamp"=w583, "ErrorSample.TxBytes"=w585, "ErrorSample.RxBytes"=w587, "ErrorSample.TxFrames"=w586) -> (w588:T1)
      }
      frame "MoveErrorCode" {
        n280 = Unbundle By Name(w592) -> ("ErrorSample"=w591:T4)
        n281 = xnode ("FIFO Method Node")("Element"=w591, "Timeout"=0) -> ()  [unwired: 1 in, 2 out]
        n282 = Bundle By Name(cluster=w592, "State"=WindSensorSampleSensorLoopStates."ClearRxFIFO") -> (w593:T1)
      }
      frame "ClearRxFIFO" {
        n283 = xnode ("FIFO Method Node")("Element"=TRUE, "Timeout"=0) -> ()  [unwired: 1 in, 2 out]
        n284 = Bundle By Name(cluster=w597, "State"=WindSensorSampleSensorLoopStates."WaitForClearComplete") -> (w598:T1)
      }
      frame "WaitForClearComplete" {
        n285 = xnode ("FIFO Method Node")("Timeout"=0) -> ("Timed Out?"=w603:bool)  [unwired: 1 in, 2 out]
        n286 = Select(t=WindSensorSampleSensorLoopStates."WaitForClearComplete", s=w603, f=WindSensorSampleSensorLoopStates."WaitForData" ("State")) -> (s? t:f=w600:T2)
        n287 = Bundle By Name(cluster=w605, "State"=w600) -> (w606:T1)
      }
    }
  }
  n288 = node-c288(w2) -> ()
